vi "员工权限管理.vi"() -> ()   [LabVIEW 2011]
uses:
  <vilib>/Utility/miscctls.llb/LVRowAndColumnUnsignedTypeDef.ctl
panel:
  in  "权限修改":bool
  in  "权限查询":bool
  out "参数浏览表":string[][](table)
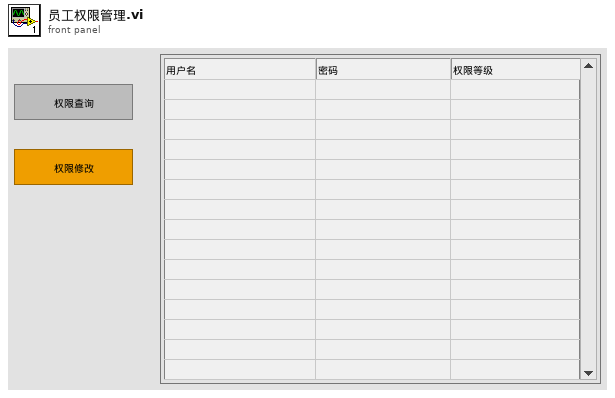
[diagram p1: front panel]
types:
  T1 = typedef "LVRowAndColumnUnsignedTypeDef.ctl" = cluster{"Row":u32, "Column":u32}
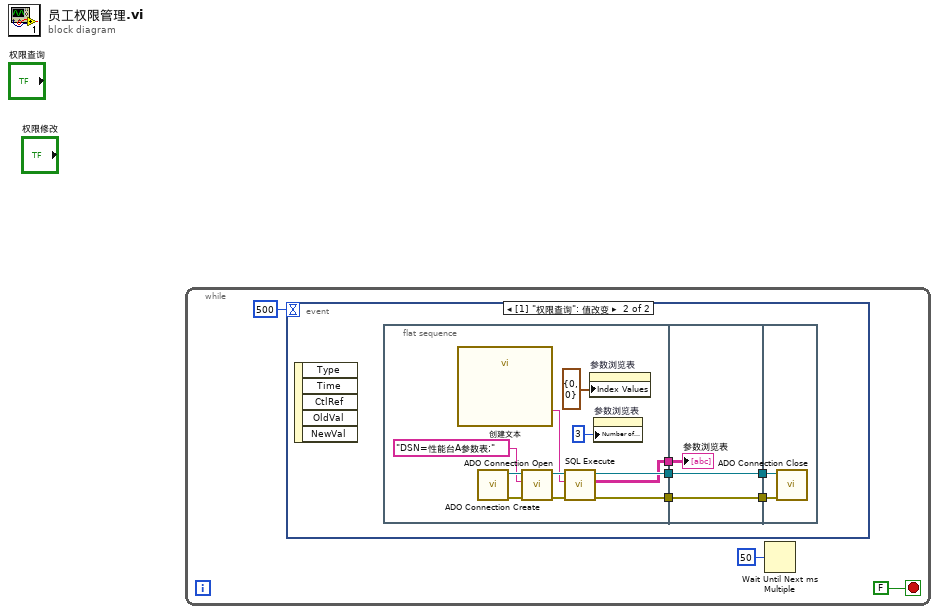
[diagram p0: block diagram]
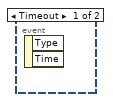
[diagram p2: hidden frame]
diagram:
  n1 = while {
    stop <- FALSE stop-if-true
    n2 = event shown="[1] \"权限查询\": 值改变" {
      selector: _ -> [_ _]
      dyn-events: _ -> [_ _]
      timeout: 500 -> [_ _]
      event Timeout {
        n3 = event-data() -> ()  [unwired: 1 in, 2 out]
      }
      event "权限查询": Value Change {
        n4 = event-data() -> ()  [unwired: 1 in, 5 out]
        n5 = flat-sequence {
          tunnel: [w11] -> w8
          tunnel: [w13] -> w7
          tunnel: [w12] -> w6
          tunnel: w8 -> [w22]
          tunnel: w7 -> [w21]
          tunnel: [w21] -> w5
          tunnel: [w20] -> w4
          tunnel: w6 -> [w20]
          tunnel: w5 -> [w24]
          tunnel: w4 -> [w23]
          frame #0 {
            n6 = call "创建文本"() -> ("Result"=w14:string)  [unwired: 14 in, 1 out]
            n7 = call "ADO Connection Create.vi"() -> ("error out"=w15:errorcluster, "ADODB._Connection Out"=w18:refnum<k7>)  [unwired: 10 in]
            n8 = call "ADO Connection Open.vi"("error in (no error)"=w15, "ConnectionString"="DSN=性能台A参数表;", "ADODB._Connection In"=w18) -> ("error out"=w19:errorcluster, "ADODB._Connection Out"=w17:refnum<k7>)  [unwired: 7 in]
            n9 = call "SQL Execute.vi"("error in (no error)"=w19, "Command Text"=w14, "ADODB._Connection In"=w17) -> ("error out"=w12:errorcluster, "Data"=w11:string[][], "ADODB._Connection Out"=w13:refnum<k7>)  [unwired: 5 in, 1 out]
            n10 = property on="参数浏览表" class="Tbl (严格)"("Index Values"=T1 {"Row"=0, "Column"=0} ("索引值")) -> ()  [unwired: 2 in, 2 out]
            n11 = property on="参数浏览表" class="Tbl (严格)"("Number of Columns"=u32 3 ("列数")) -> ()  [unwired: 2 in, 2 out]
          }
          frame #1 {
            "参数浏览表" <- w22
          }
          frame #2 {
            n12 = call "ADO Connection Close.vi"("error in (no error)"=w23, "ADODB._Connection In"=w24) -> ()  [unwired: 8 in, 2 out]
          }
        }
      }
    }
    n13 = Wait Until Next ms Multiple(millisecond multiple=u32 50 ("毫秒倍数")) -> ()  [unwired: 1 out]
  }
